vi "Ej_9_Filtro_EMA.vi"() -> ()   [LabVIEW 2021]
panel:
  out "appended array":dbl[](array[numeric])
  in  "Array":dbl[](array[numeric])
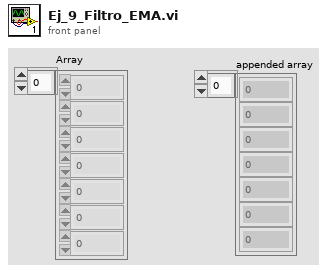
[diagram p1: front panel]
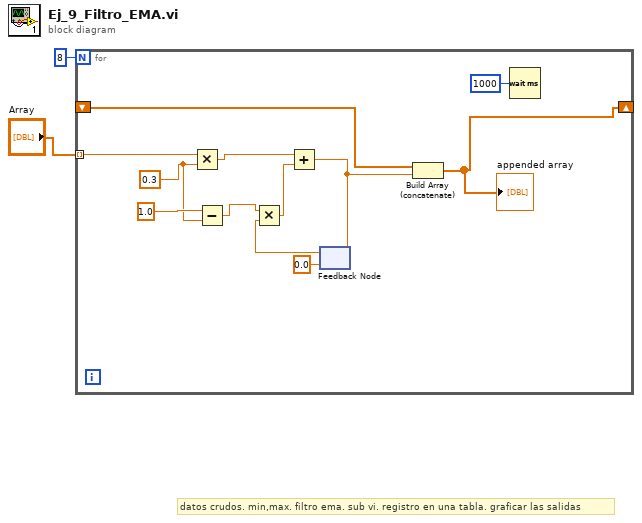
[diagram p0: block diagram]
diagram:
  # "datos crudos. min,max. filtro ema. sub vi. registro en una tabla. graficar las salidas"
  n1 = for {
    N: 8 -> [_]
    tunnel: "Array" -> [w6] mode=indexing
    shift-right: [w3] -> _
    shift-left: _ -> [w4]
    w10 = 0.3 ("y")
    n2 = Multiply(x=w6, y=w10) -> (x*y=w14:dbl)
    n3 = Subtract(x=1.0, y=w10) -> (x-y=w12:dbl)
    n4 = feedback #1(0.0) -> (w9:dbl)
    n5 = Multiply(x=w12, y=w9) -> (x*y=w13:dbl)
    n6 = Add(x=w14, y=w13) -> (x+y=w7:dbl)
    n7 = feedback-in #1(w7) -> ()
    n8 = Build Array (concatenate)(w4, w7) -> (w3:dbl[])
    "appended array" <- w3
    n9 = Wait (ms)(milliseconds to wait=u32 1000) -> ()  [unwired: 1 out]
  }
